vi "SendSetLogDirectory.vi"(8 "error in (no error)":errorcluster, 9 "tracpoint directory":path, 10 "log directory":path, 11 "qbus in":refnum<class "Qbus.lvclass">) -> (0 "error out":errorcluster, 3 "qbus out":refnum<class "Qbus.lvclass">)   [LabVIEW 2017, in "TraceLogger.lvlib"]
uses:
  <vilib>/addons/TraceLogger/TraceLogger.lvlib
  <vilib>/addons/Qbus/Qbus.lvclass
  <vilib>/addons/TraceLogger/controls/TracpointDirectories.ctl
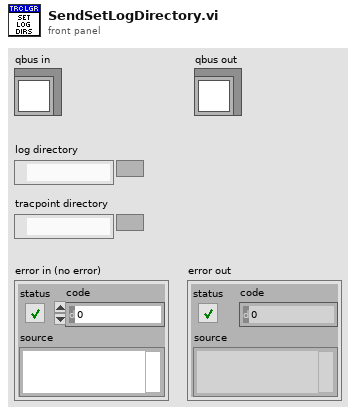
[diagram p1: front panel]
types:
  T1 = typedef "TracpointDirectories.ctl" = cluster{"log directory":path, "tracpoint directory":path}
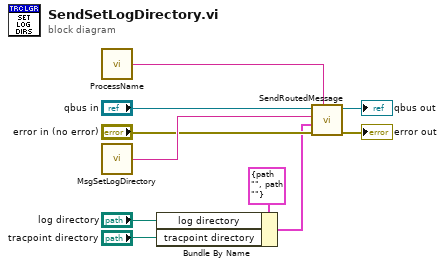
[diagram p0: block diagram]
diagram:
  n1 = call <vilib>:"ProcessName.vi"() -> ("process name"=w6:string)  [unwired: 5 in]
  n2 = call <vilib>:"MsgSetLogDirectory.vi"() -> ("message name"=w7:string)  [unwired: 5 in]
  n3 = Bundle By Name(cluster=T1 {"log directory"=path "", "tracpoint directory"=path ""} ("tracpoint directories"), "log directory"="log directory", "tracpoint directory"="tracpoint directory") -> (w3:T1)
  n4 = call <vilib>:"SendRoutedMessage.vi"("listener process"=w6, "error in (no error)"="error in (no error)", "message value"=w3, "message name"=w7, "Qbus in"="qbus in") -> ("error in (no error)"=→"error out":errorcluster, "Qbus out"=→"qbus out":refnum<class "Qbus.lvclass">)  [unwired: 5 in]
